vi "WaitData.vi"(8 "error in (no error)":errorcluster, 10 "Timeout":dbl, 11 "VISA Refnum in":refnum<visa-resource-name>) -> (0 "error out":errorcluster, 2 "Device Status":i32 format="%04x", 3 "VISA Refnum out":refnum<visa-resource-name>, 5 "OK?":bool)   [LabVIEW 2020]
doc: "This VI queries the status of the device and evaluates if the data are ready to be acquired or not.\nIf timeout expires before the data are ready, the OK? indicator value will be FALSE"
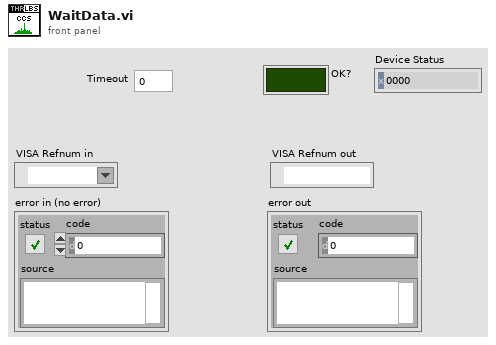
[diagram p1: front panel]
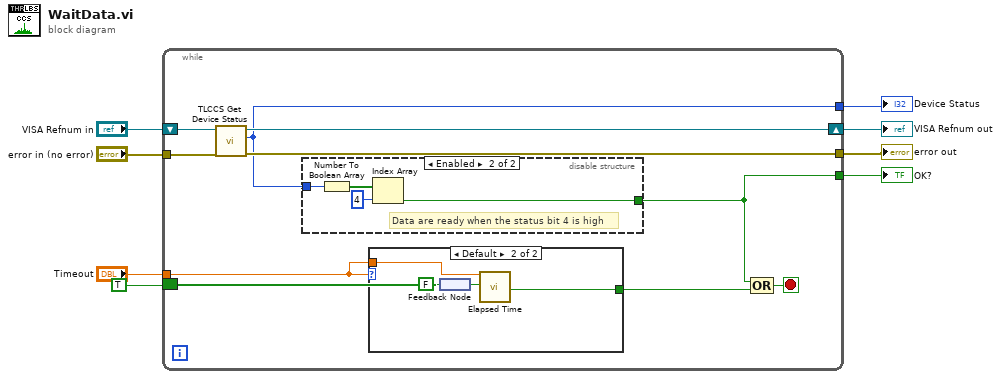
[diagram p0: block diagram]
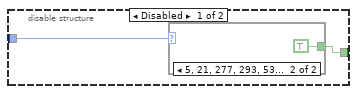
[diagram p2: hidden frame]
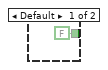
[diagram p3: hidden frame]
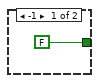
[diagram p4: hidden frame]
diagram:
  n1 = while {
    tunnel: "error in (no error)" -> [w16]
    tunnel: [w15] -> w7
    tunnel: "Timeout" -> [w9]
    border: TRUE -> [_]
    tunnel: [w10] -> w2
    tunnel: [w11] -> w1
    shift-right: [w14] -> w8
    shift-left: "VISA Refnum in" -> [w17]
    stop <- w12 stop-if-true
    n2 = call <instrlib>:"TLCCS Get Device Status.vi"("error in (no error)"=w16, "instrument handle"=w17) -> ("error out"=w15:errorcluster, "Device Status"=w11:i32, "instrument handle out"=w14:refnum<visa-resource-name>)  [unwired: 7 in]
    n3 = disable-structure shown="Enabled" {
      disable-tunnel: w11 -> [w19 w25]
      disable-tunnel: [w18 w22] -> w10
      frame Disabled {
        n4 = case shown="5, 21, 277, 293, 533, 789" w19 {
          tunnel: [FALSE TRUE] -> w18
          frame Default {
          }
          frame 5, 21, 277, 293, 533, 789 {
          }
        }
      }
      frame Enabled {
        # "Data are ready when the status bit 4 is high"
        n5 = Number To Boolean Array(number=w25) -> (Boolean array=w24:bool[])
        n6 = Index Array(array=w24, index=4) -> (element=w22:bool)
      }
    }
    n7 = case shown="Default" w9 {
      tunnel: [FALSE ("Time has Elapsed") w28] -> w13
      tunnel: w9 -> [_ w27]
      frame -1 {
      }
      frame Default {
        n8 = feedback #1() -> (w30:bool)
        n9 = feedback-in #1(FALSE) -> ()
        n10 = call "Elapsed Time"("Time Target (s)"=w27, "Reset"=w30) -> ("Time has Elapsed"=w28:bool)  [unwired: 10 in, 7 out]
      }
    }
    n11 = Compound Arithmetic op=OR(w10, w13) -> (w12:bool)
  }
  "VISA Refnum out" <- w8
  "error out" <- w7
  "OK?" <- w2
  "Device Status" <- w1
